vi "Configure Output Characteristics.vi"(7 "Item (1)":i32=1 min=1 max=255 step=1, 8 "error in (no error)":errorcluster, 10 "Function (Empty)":string, 11 "VISA resource name":refnum<visa-resource-name>) -> (0 "error out":errorcluster, 3 "VISA resource name out":refnum<visa-resource-name>)   [LabVIEW 2020, in "Yokogawa WT300 Series.lvlib"]
doc: "Configures the normal numeric features."
uses:
  Yokogawa WT300 Series.lvlib
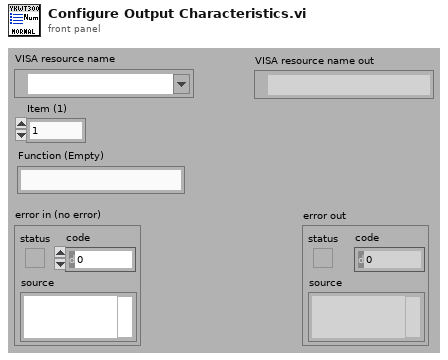
[diagram p1: front panel]
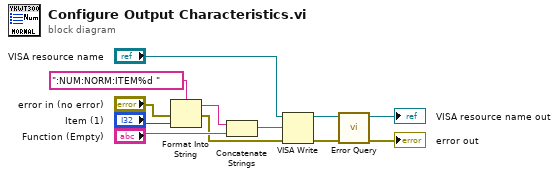
[diagram p0: block diagram]
diagram:
  n1 = Format Into String(format string=":NUM:NORM:ITEM%d " ("形式文字列"), error in="error in (no error)", "Item (1)") -> (resulting string=w4:string, error out=w2:errorcluster)  [unwired: 1 in]
  n2 = Concatenate Strings(w4, "Function (Empty)") -> (w1:string)
  n3 = VISA Write ("VISA書き込み")(VISA resource name="VISA resource name", write buffer=w1, error in (no error)=w2) -> (VISA resource name out=w12:refnum<visa-resource-name>, error out=w11:errorcluster)  [unwired: 1 out]
  n4 = call "Error Query.vi"("error in (no error)"=w11, "VISA resource name"=w12) -> ("error out"=→"error out":errorcluster, "VISA resource name out"=→"VISA resource name out":refnum<visa-resource-name>)  [unwired: 6 in, 2 out]
